vi "uService GUI.vi"(8 "error in (no error)":errorcluster, 11 "uService Template in":refnum<class "DAQ Manager.lvclass">) -> (3 "uService Template out":refnum<class "DAQ Manager.lvclass">)   [LabVIEW 2020, in "TALOS.lvlib" / "DAQ Manager.lvlib" / "DAQ Manager.lvclass"]
uses:
  DAQ Manager.lvclass
  C:/LabVIEW Code/TALOS/talos/Father of all uServices/Father of all uServices/Father of all uServices.lvclass
  Ancestor/Ancestor/Ancestor.lvclass/Ancestor.ctl
  Support VIs/Substitute Error.vi
  Support VIs/Generate Error.vi
  FGV/Error Memory/Get Error Description.vi
  Support VIs/Get PC name.vi
  Ancestor/Ancestor/Read ID.vi
  Support VIs/Get Class Name.vi
  FGV/Error Memory/Error Memory Core.vi
  <vilib>/AdvancedString/Delimited String to 1D String Array.vi
  Support VIs/Circus Root Path.vi
  FGV/Error Memory/Error Crt Lvl checker.vi
  FGV/Error Memory/Error Memory Core.vi/40c8088d-b597-4017-91af-faa98e00292e.vi
  FGV/Error Memory/Error Memory Core.vi/d4a3ab98-063c-4e44-b43d-fbdcfe6c2be2.vi
  Father of all uServices/Father of all uServices/Father of all uServices.lvclass
  C:/LabVIEW Code/TALOS/builds/Actor Framework PPL/Actor Framework.lvlibp/1abvi3w/vi.lib/ActorFramework/Actor/Actor.lvclass
  builds/Actor Framework PPL/Actor Framework.lvlibp/1abvi3w/vi.lib/ActorFramework/Actor/Read Self Enqueuer.vi
  builds/Actor Framework PPL/Actor Framework.lvlibp/1abvi3w/vi.lib/ActorFramework/Stop Msg/Send Normal Stop.vi
  Support VIs/Global Memory.vi
  <vilib>/Utility/LVClass/Get LV Class Name.vi
  Support VIs/Is in Packed Library.vi
  Support VIs/TALOS Root path.vi
  Support VIs/Read CSV worksheet.vi
  Support VIs/Global Constants.vi
  <vilib>/Utility/error.llb/General Error Handler.vi
  Support VIs/Error Log.vi
  Ancestor/Ancestor/Ancestor.lvclass
  <vilib>/Comparison/Equal/Equal Functor/Equal Functor.lvclass
panel:
  out "Closure duration":dbl
  in  "Test send DAQ":bool
  out "RUN Path":string
  out "RUN Port":u16
  out "RUN Number":u32
  out "RUN Active":bool
  in  "Stop Run":bool
  in  "Get Run Status":bool
  in  "stop New uService":bool
  in  "Start Run":bool
  # "DAQ Manager"
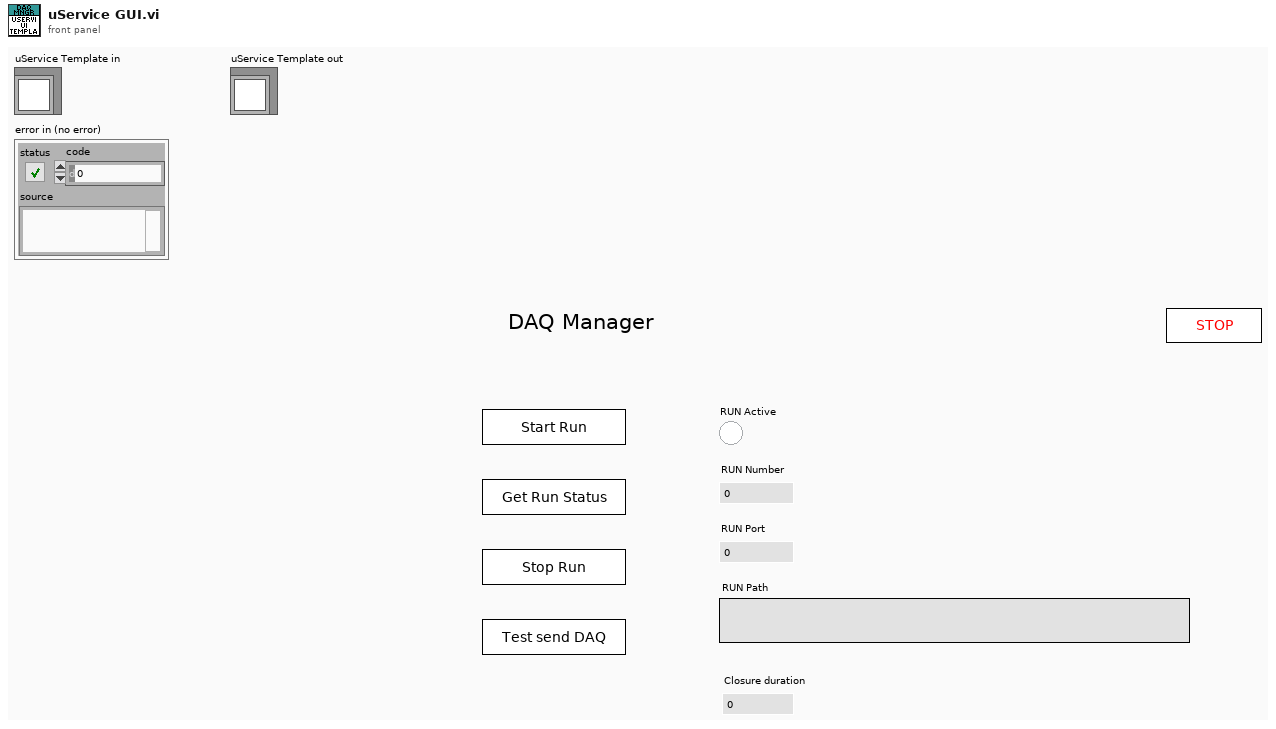
[diagram p1: front panel]
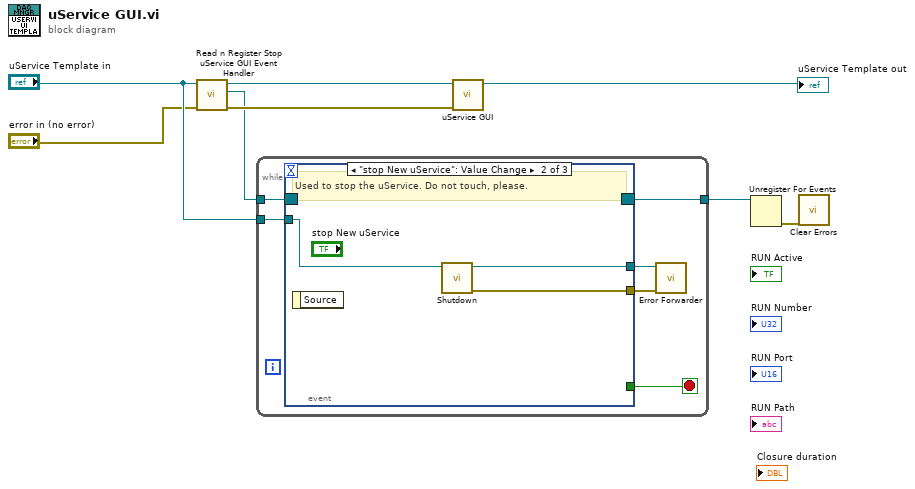
[diagram p0: block diagram]
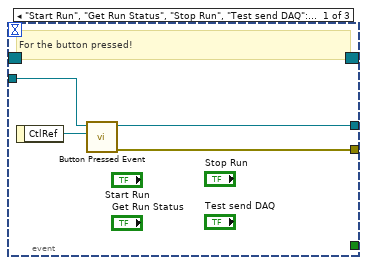
[diagram p2: hidden frame]
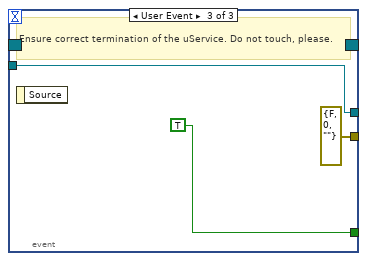
[diagram p3: hidden frame]
diagram:
  n1 = call-dynamic "Read n Register Stop uService GUI Event Handler .vi"("error in (no error)"="error in (no error)", "uService Template in"="uService Template in") -> ("error out"=w6:errorcluster, "Stop uService GUI Event Ref"=w5:refnum<event-registration>, "uService Template out"=w7:refnum<class "DAQ Manager.lvclass">)  [unwired: 7 in]
  n2 = while {
    tunnel: [w14] -> w8
    tunnel: w5 -> [w12]
    tunnel: "uService Template in" -> [w11]
    stop <- w13 stop-if-true
    n3 = event shown="[1] \"stop New uService\": Value Change" {
      selector: w12 -> [_ _ _]
      dyn-events: [_ _ _] -> w14
      timeout: _ -> [_ _ _]
      tunnel: [_ _ TRUE] -> w13
      tunnel: w11 -> [w18 w21 w23]
      tunnel: [w15 w20 errorcluster {"status"=FALSE, "code"=0, "source"=""} ("error out")] -> w10
      tunnel: [w16 w19 w23] -> w9
      event "Start Run", "Get Run Status", "Stop Run", "Test send DAQ": Value Change {
        # "For the button pressed!"
        n4 = event-data() -> ("CtlRef"=w17:refnum<vi>)  [unwired: 1 in]
        n5 = call-dynamic "Button Pressed Event.vi"("CtlRef"=w17, "uService Template in"=w18) -> ("error out"=w15:errorcluster, "uService Template out"=w16:refnum<class "DAQ Manager.lvclass">)  [unwired: 8 in]
      }
      event "stop New uService": Value Change {
        # "Used to stop the uService. Do not touch, please."
        n6 = event-data() -> ()  [unwired: 1 in, 1 out]
        n7 = call "Shutdown.vi"("Father of all uServices in"=w21) -> ("error out"=w20:errorcluster, "Father of all uServices out"=w19:refnum<class "DAQ Manager.lvclass">)  [unwired: 9 in]
      }
      event User Event {
        # "Ensure correct termination of the uService. Do not touch, please."
        n8 = event-data() -> ()  [unwired: 1 in, 1 out]
      }
    }
    n9 = call "Error Forwarder.vi"("error in (no error)"=w10, "Father of all uServices in"=w9) -> ()  [unwired: 10 in]
  }
  n10 = call-parent "uService GUI.vi"("error in (no error)"=w6, "uService Template in"=w7) -> ("uService Template out"=→"uService Template out":refnum<class "DAQ Manager.lvclass">)  [unwired: 9 in]
  n11 = Unregister For Events(event registration refnum=w8) -> (error out=w1:errorcluster)  [unwired: 1 in]
  n12 = call <vilib>:"Clear Errors.vi"("error in (no error)"=w1) -> ()  [unwired: 5 in, 2 out]
